vi "Lock-in Globals Multiple Inputs and Outputs.vi"() -> ()   [LabVIEW 2013]
panel:
  out "Gain Cal":dbl[](array[numeric])=[1.0, 2e-08, 0.001, 0.001, 0.001, 2e-08]
  in  "Simple Average?":bool
  in  "Voltage Channels":cluster{"V+ Channel":i32, "V- Channel":i32}[](array[cluster])
  in  "Vbg":dbl=1.0
  in  "KH Channel Setting":T1(array[cluster])=[{"Channel"=1, "Gain"=4, "Shunt Resistor"=5, "Measure"=1}, {"Channel"=2, "Gain"=4, "Shunt Resistor"=1, "Measure"=2}, {"Channel"=3, "Gain"=4, "Shunt Resistor"=1, "Measure"=2}, {"Channel"=4, "Gain"=4, "Shunt Resistor"=1, "Measure"=2}, {"Channel"=5, "Gain"=4, "Shunt Resistor"=1, "Measure"=2}, {"Channel"=6, "Gain"=4, "Shunt Resistor"=5, "Measure"=1}, {"Channel"=7, "Gain"=4, "Shunt Resistor"=5, "Measure"=1}, {"Channel"=8, "Gain"=4, "Shunt Resistor"=5, "Measure"=1}] {"Measure" items=["Float", "Current(Diff)", "Voltage(SE+)"]; "Shunt Resistor" items=["Open"=1, "50 Ohms"=2, "500 Ohms"=3, "5k Ohms"=4, "50k Ohms"=5]; "Gain" items=["1x"=1, "10x"=2, "100x"=3, "1000x"=4]; "Channel" items=["Channel 1"=1, "Channel 2"=2, "Channel 3"=3, "Channel 4"=4, "Channel 5"=5, "Channel 6"=6, "Channel 7"=7, "Channel 8"=8]}
  in  "VH+ Channel":i32=1
  in  "VH- Channel":i32=2
  in  "Source- Card#":i32
  in  "Source- AO#":i32
  in  "Source- Channel":i32=1
  in  "1D OSC Configuration":T2(array[cluster])=[{"Signal Type"=enum."Sine Wave", "DC"=0.0, "Amplitude"=0.0, "frequency"=1.0, "Phase"=0.0}, {"Signal Type"=enum."Sine Wave", "DC"=0.0, "Amplitude"=0.0, "frequency"=1.346, "Phase"=0.0}, {"Signal Type"=enum."Sine Wave", "DC"=0.0, "Amplitude"=0.0, "frequency"=1.346, "Phase"=0.0}, {"Signal Type"=enum."Sine Wave", "DC"=0.0, "Amplitude"=0.0, "frequency"=1.346, "Phase"=0.0}, {"Signal Type"=enum."Sine Wave", "DC"=0.0, "Amplitude"=0.0, "frequency"=1.346, "Phase"=0.0}, {"Signal Type"=enum."Sine Wave", "DC"=0.0, "Amplitude"=0.001, "frequency"=1.346, "Phase"=0.0}, {"Signal Type"=enum."Sine Wave", "DC"=0.0, "Amplitude"=0.0, "frequency"=1.346, "Phase"=0.0}, {"Signal Type"=enum."Sine Wave", "DC"=0.0, "Amplitude"=0.0, "frequency"=1.346, "Phase"=0.0}, {"Signal Type"=enum."Sine Wave", "DC"=0.0, "Amplitude"=0.0, "frequency"=1.346, "Phase"=0.0}] {"frequency" step=0.001 format="%.3p"; "Amplitude" format="%0.2p"; "DC" min=-0.99 max=0.99 format="%.2p"}
  in  "Sidegate Channel":i32=3
  in  "Source Channel":i32=1
  out "Remote Stop Lockin":bool
  in  "Sidegate AO#":i32=1
  in  "Sidegate Card#":i32
  in  "Source Card#":i32
  in  "V+ Channel":i32=1
  in  "V- Channel":i32=2
  in  "Current Channel":i32
  in  "Source AO#":i32
  out "Timestamp":timestamp
  out "1/Gain":dbl[](array[numeric])=[1.0, 2e-08, 0.001, 0.001, 0.001, 2e-08]
  out "Output":waveform(dbl)[][](array[waveform])
  in  "Sampling information":cluster{"Fs":dbl, "#s":dbl}[](array[cluster])=[{"Fs"=100000.0, "#s"=200000.0}, {"Fs"=100000.0, "#s"=200000.0}]
  out "Reset Lockin":bool
  in  "Multiplication factor":dbl=1.0
  out "DAQ Input signal":dbl[][](graph)
  out "Stop Lockin":bool
  out "Results":dbl[][](array[numeric])=[[1.4839408729757508e-11, -1.900879392885926e-12, 1.4960661546706472e-11, -7.299647829275913], [1.7200124080450918e-16, -5.0346392409039706e-17, 1.7921826376487348e-16, -16.315253344298398], [1.1117395670783847e-11, -2.59351111233741e-11, 2.8217485279211652e-11, -66.79702725745167], [-3.930657765785384e-11, 1.8195590831737717e-12, 3.934867014817724e-11, 177.3495865094821]]
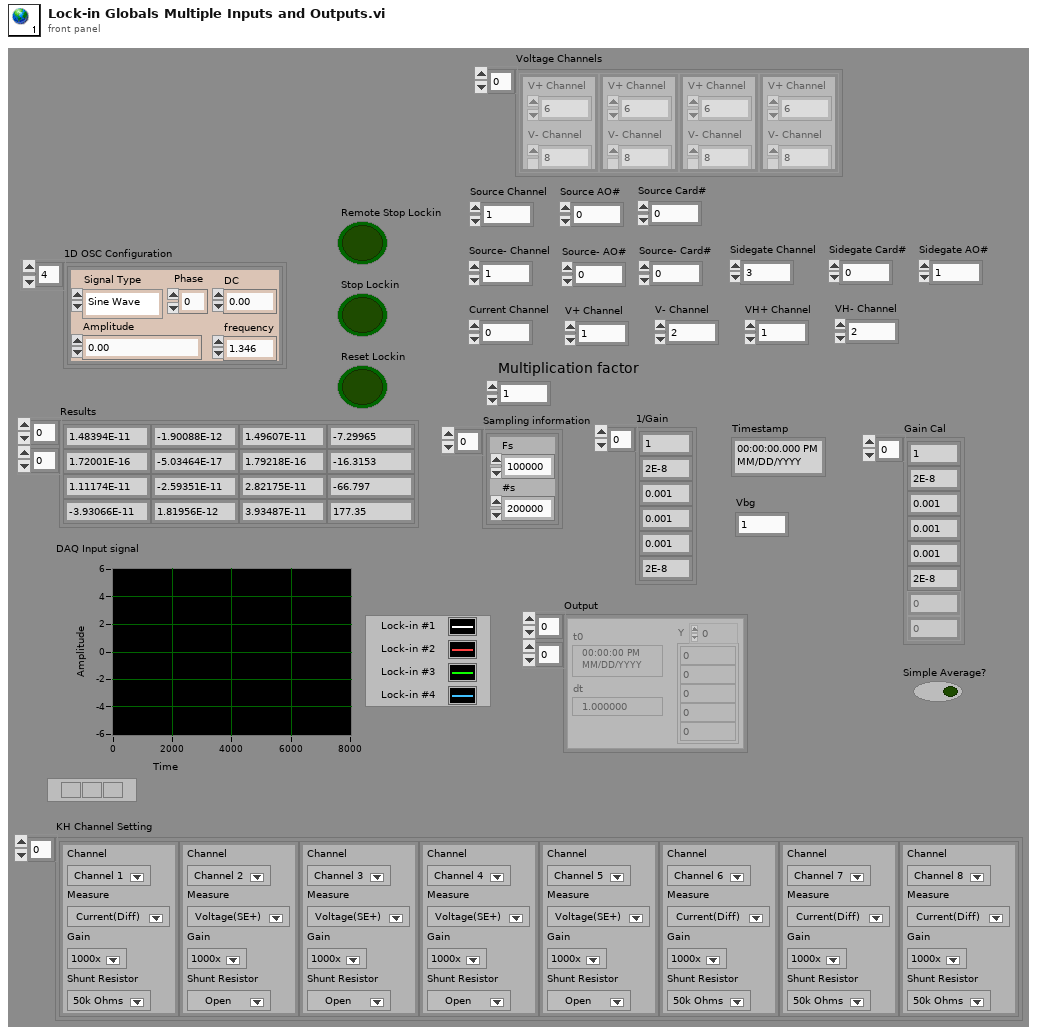
[diagram p1: front panel]
types:
  T1 = cluster{"Channel":u16, "Gain":u16, "Shunt Resistor":u16, "Measure":u16}[]
  T2 = cluster{"Signal Type":enum16{"Sine Wave", "Triangle Wave", "Square Wave", "Sawtooth Wave"}, "DC":dbl, "Amplitude":dbl, "frequency":dbl, "Phase":dbl}[]
diagram:
